vi "SiosIfmGetTriggerSettings.vi"(0 "devNumber":i32) -> (1 "success":i32, 2 "TriggerSettings":T1)   [LabVIEW 2009]
uses:
  siosifm.dll
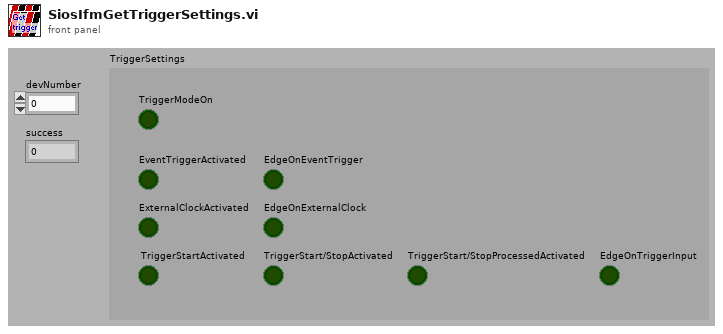
[diagram p1: front panel]
types:
  T1 = cluster{"TriggerModeOn":bool, "EventTriggerActivated":bool, "EdgeOnEventTrigger":bool, "ExternalClockActivated":bool, "EdgeOnExternalClock":bool, "TriggerStartActivated":bool, "TriggerStart/StopActivated":bool, "TriggerStart/StopProcessedActivated":bool, "EdgeOnTriggerInput":bool}
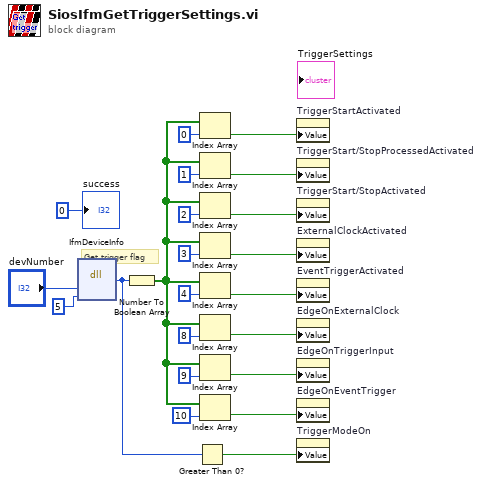
[diagram p0: block diagram]
diagram:
  # "Get trigger flag"
  n1 = dll-call lib="D:/Support/Labview/RE-10/SIOS_IfmDLL/siosifm.dll" fn="IfmDeviceInfo"("devNumber"="devNumber", "requestedInfoFlag"=u32 5) -> (w2:u32)  [unwired: 5 in, 2 out]
  n2 = Number To Boolean Array(number=w2) -> (Boolean array=w7:bool[])
  n3 = Greater Than 0?(x=w2) -> (x > 0?=w3:bool)
  n4 = Index Array(array=w7, index=0 ("Index")) -> (element=w22:bool)
  n5 = Index Array(array=w7, index=1 ("Index")) -> (element=w21:bool)
  n6 = Index Array(array=w7, index=2 ("Index")) -> (element=w20:bool)
  n7 = Index Array(array=w7, index=3 ("Index")) -> (element=w19:bool)
  n8 = Index Array(array=w7, index=4 ("Index")) -> (element=w18:bool)
  n9 = Index Array(array=w7, index=8 ("Index")) -> (element=w6:bool)
  n10 = Index Array(array=w7, index=9 ("Index")) -> (element=w5:bool)
  n11 = Index Array(array=w7, index=10 ("Index")) -> (element=w4:bool)
  n12 = property on="TriggerStartActivated" class="Boolesch (strikt)"("Value"=w22) -> ()  [unwired: 2 in, 2 out]
  n13 = property on="TriggerStart/StopProcessedActivated" class="Boolesch (strikt)"("Value"=w21) -> ()  [unwired: 2 in, 2 out]
  n14 = property on="TriggerStart/StopActivated" class="Boolesch (strikt)"("Value"=w20) -> ()  [unwired: 2 in, 2 out]
  n15 = property on="ExternalClockActivated" class="Boolesch (strikt)"("Value"=w19) -> ()  [unwired: 2 in, 2 out]
  n16 = property on="EventTriggerActivated" class="Boolesch (strikt)"("Value"=w18) -> ()  [unwired: 2 in, 2 out]
  n17 = property on="EdgeOnExternalClock" class="Boolesch (strikt)"("Value"=w6) -> ()  [unwired: 2 in, 2 out]
  n18 = property on="EdgeOnTriggerInput" class="Boolesch (strikt)"("Value"=w5) -> ()  [unwired: 2 in, 2 out]
  n19 = property on="EdgeOnEventTrigger" class="Boolesch (strikt)"("Value"=w4) -> ()  [unwired: 2 in, 2 out]
  n20 = property on="TriggerModeOn" class="Boolesch (strikt)"("Value"=w3) -> ()  [unwired: 2 in, 2 out]
  "success" <- 0
